vi "Wait-for-start.vi"(8 "error in":errorcluster, 10 "UI ref. in":refnum<data-value>, 11 "Data ref. in":refnum<data-value>) -> (0 "error IO":errorcluster, 2 "UI ref.":refnum<data-value>, 3 "Data ref.":refnum<data-value>, 5 "Proceed?":bool)   [LabVIEW 2013, in "CameraVision.lvlib" / "CV-Main.lvclass"]
doc: "If the acquisition start option is 'Post-phoned', this function will pause the operation untill the specified start time is reached. The timing is accurate to 1 second.\nIn case the specified start time is in the past, the acquisition is started immediately.\nIf the 'Stop' button is pressed or the window is closed before the start time is reached, the operation is aborted."
uses:
  CV-Main.lvclass
  UI/CV-UI.lvclass
  UI/CV-UI.lvclass/CV-UI.ctl
  CV-Main.lvclass/CV-Main.ctl
  Acquisition/CV-Acquisition.lvclass/CV-Acquisition.ctl
  Acquisition/Read Acquisition start.vi
  Acquisition/Read Start time.vi
  Read Acquis params.vi
  UI/Read Acquisition.vi
  Acquisition/CV-Acquisition.lvclass
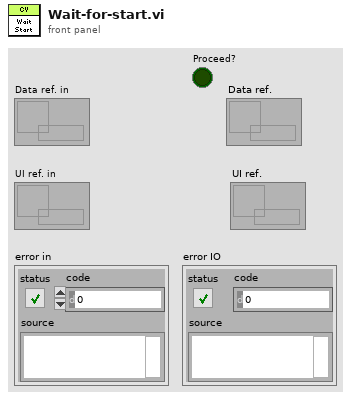
[diagram p1: front panel]
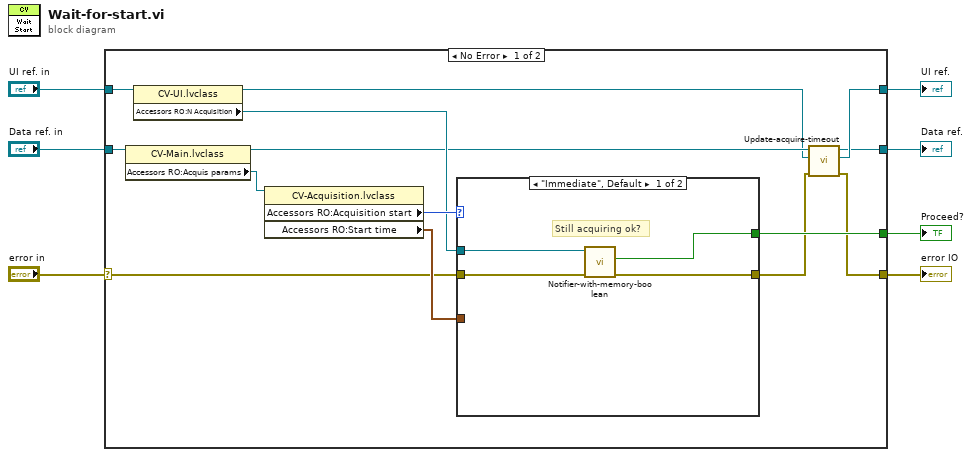
[diagram p0: block diagram]
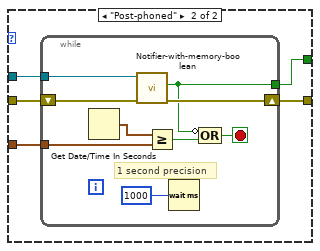
[diagram p2: hidden frame]
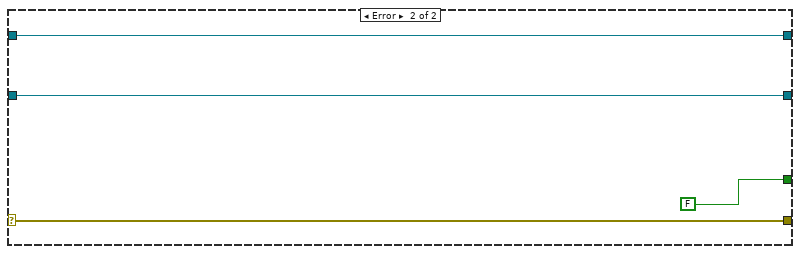
[diagram p3: hidden frame]
diagram:
  n1 = case shown="No Error" "error in" {
    selector: "error in" -> [w15 w43]
    tunnel: [w10 w43] -> w7
    tunnel: [w21 FALSE] -> w5
    tunnel: "Data ref. in" -> [w18 w40]
    tunnel: "UI ref. in" -> [w17 w41]
    tunnel: [w8 w40] -> w2
    tunnel: [w12 w41] -> w1
    frame No Error {
      n2 = property class="CV-Main.lvclass"(reference=w18) -> (reference out=w13:refnum<data-value>, "Accessors RO:Acquis params"=w16:refnum<data-value>)  [unwired: 1 in, 1 out]
      n3 = property class="CV-UI.lvclass"(reference=w17) -> (reference out=w11:refnum<data-value>, "Accessors RO:N Acquisition"=w14:refnum<notifier>)  [unwired: 1 in, 1 out]
      n4 = property class="CV-Acquisition.lvclass"(reference=w16) -> ("Accessors RO:Acquisition start"=w20:enum16{"Immediate", "Post-phoned"}, "Accessors RO:Start time"=w19:timestamp)  [unwired: 1 in, 2 out]
      n5 = case shown="\"Immediate\", Default" w20 {
        tunnel: w15 -> [w24 w30]
        tunnel: [w23 w26] -> w9
        tunnel: w19 -> [_ w29]
        tunnel: w14 -> [w25 w28]
        tunnel: [w22 w27] -> w21
        frame "Immediate", Default {
          # "Still acquiring ok?"
          n6 = call "Notifier-with-memory-boolean.vi"("error in"=w24, "Notifier in"=w25) -> ("error IO"=w23:errorcluster, "Notification"=w22:bool)  [unwired: 8 in]
        }
        frame "Post-phoned" {
          n7 = while {
            shift-right: [w32] -> w26
            shift-left: w30 -> [w33]
            tunnel: w29 -> [w38]
            tunnel: w28 -> [w34]
            tunnel: [w31] -> w27
            stop <- w37 stop-if-true
            # "1 second precision"
            n8 = Get Date/Time In Seconds() -> (seconds since 1Jan1904=w35:timestamp)
            n9 = call "Notifier-with-memory-boolean.vi"("error in"=w33, "Notifier in"=w34) -> ("error IO"=w32:errorcluster, "Notification"=w31:bool)  [unwired: 8 in]
            n10 = Greater Or Equal?(x=w35, y=w38) -> (x >= y?=w36:bool)
            n11 = Wait (ms)(milliseconds to wait=u32 1000) -> ()  [unwired: 1 out]
            n12 = Compound Arithmetic op=OR(invert w31, w36) -> (w37:bool)
          }
        }
      }
      n13 = call "Update-acquire-timeout.vi"("error in"=w9, "UI ref. in"=w11, "Data ref. in"=w13) -> ("error IO"=w10:errorcluster, "UI ref."=w12:refnum<data-value>, "Data ref."=w8:refnum<data-value>)  [unwired: 6 in]
    }
    frame Error {
    }
  }
  "error IO" <- w7
  "Proceed?" <- w5
  "UI ref." <- w1
  "Data ref." <- w2
